vi "Test Bool.vi"() -> ()   [LabVIEW 2021]
uses:
  Source/Bool/Initialise.vi
  Source/Bool/conc_SharedVar_Bool.lvclass
panel:
  in  "stop":bool
  out "Boolean 2":bool
  in  "Boolean":bool
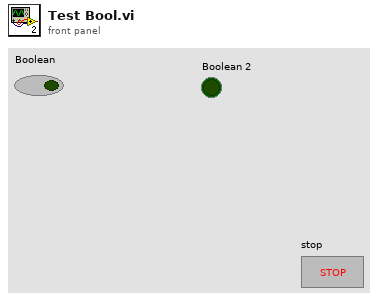
[diagram p1: front panel]
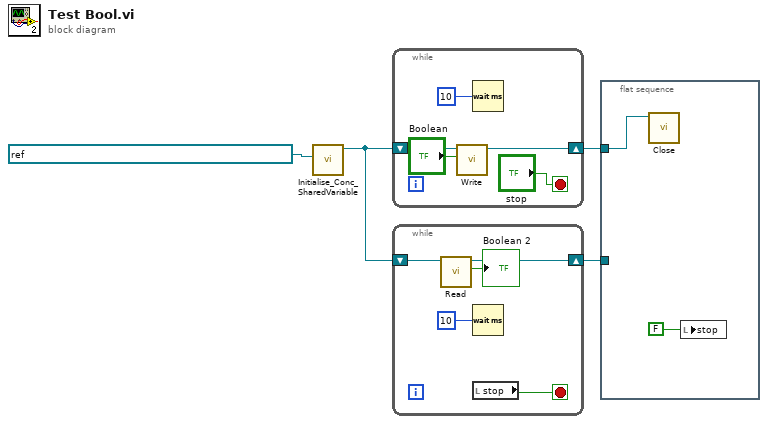
[diagram p0: block diagram]
diagram:
  n1 = call-poly "Initialise_Conc_SharedVariable.vi"("shared variable refnum"=refnum<k21> "ni.var.psp://localhost/Test Shared Variables/Bool") -> ("abs_SharedVar_Bool out"=w2:refnum<class "conc_SharedVar_Bool.lvclass">)  [unwired: 9 in, 1 out]
  n2 = while {
    shift-right: [w9] -> w4
    shift-left: w2 -> [w8]
    stop <- "stop" stop-if-true
    n3 = call-dynamic "Write.vi"("Boolean"="Boolean", "Boolean in"=w8) -> ("Boolean out"=w9:refnum<class "conc_SharedVar_Bool.lvclass">)  [unwired: 8 in, 1 out]
    n4 = Wait (ms)(milliseconds to wait=u32 10) -> ()  [unwired: 1 out]
  }
  n5 = while {
    shift-right: [w13] -> w3
    shift-left: w2 -> [w14]
    stop <- w10 stop-if-true
    n6 = call-dynamic "Read.vi"("Boolean in"=w14) -> ("Boolean"=→"Boolean 2":bool, "Boolean out"=w13:refnum<class "conc_SharedVar_Bool.lvclass">)  [unwired: 8 in, 1 out]
    n7 = Wait (ms)(milliseconds to wait=u32 10) -> ()  [unwired: 1 out]
    n8 = local read "stop"() -> (w10:bool)
  }
  n9 = flat-sequence {
    tunnel: w4 -> [w16]
    tunnel: w3 -> [_]
    frame #0 {
      n10 = call-dynamic "Close.vi"("Data in"=w16) -> ()  [unwired: 9 in, 2 out]
      n11 = local write "stop"(FALSE ("stop")) -> ()
    }
  }
